vi "globalArrows.vi"() -> ()   [LabVIEW 2020]
panel:
  out "empty":u32[][](array[colorbox])=[[0, 0, 0, 0, 0, 0, 0, 0], [0, 0, 0, 0, 0, 0, 0, 0], [0, 0, 0, 0, 0, 0, 0, 0], [0, 0, 0, 0, 0, 0, 0, 0], [0, 0, 0, 0, 0, 0, 0, 0], [0, 0, 0, 0, 0, 0, 0, 0], [0, 0, 0, 0, 0, 0, 0, 0], [0, 0, 0, 0, 0, 0, 0, 16777222]]
  out "left":u32[][](array[colorbox])=[[0, 0, 0, 0, 0, 0, 0, 0], [0, 0, 6618880, 0, 0, 0, 0, 0], [0, 6618880, 0, 0, 0, 0, 0, 0], [6618880, 6618880, 6618880, 6618880, 6618880, 6618880, 0, 0], [0, 6618880, 0, 0, 0, 0, 0, 0], [0, 0, 6618880, 0, 0, 0, 0, 0], [0, 0, 0, 0, 0, 0, 0, 0], [16777222, 0, 0, 0, 0, 0, 0, 0]]
  out "up":u32[][](array[colorbox])=[[0, 0, 0, 6618880, 0, 0, 0, 16777222], [0, 0, 6618880, 6618880, 6618880, 0, 0, 0], [0, 6618880, 0, 6618880, 0, 6618880, 0, 0], [0, 0, 0, 6618880, 0, 0, 0, 0], [0, 0, 0, 6618880, 0, 0, 0, 0], [0, 0, 0, 6618880, 0, 0, 0, 0], [0, 0, 0, 0, 0, 0, 0, 0], [0, 0, 0, 0, 0, 0, 0, 0]]
  out "down":u32[][](array[colorbox])=[[0, 0, 0, 0, 0, 0, 0, 0], [0, 0, 0, 0, 0, 0, 0, 0], [0, 0, 0, 6618880, 0, 0, 0, 0], [0, 0, 0, 6618880, 0, 0, 0, 0], [0, 0, 0, 6618880, 0, 0, 0, 0], [0, 6618880, 0, 6618880, 0, 6618880, 0, 0], [0, 0, 6618880, 6618880, 6618880, 0, 0, 0], [0, 0, 0, 6618880, 0, 0, 0, 16777222]]
  out "enter":u32[][](array[colorbox])=[[0, 0, 0, 0, 0, 0, 6618880, 0], [0, 0, 6618880, 0, 0, 0, 6618880, 0], [0, 6618880, 0, 0, 0, 0, 6618880, 0], [6618880, 6618880, 6618880, 6618880, 6618880, 6618880, 6618880, 0], [0, 6618880, 0, 0, 0, 0, 0, 0], [0, 16777222, 6618880, 0, 0, 0, 0, 0], [0, 0, 16777222, 0, 0, 0, 0, 0], [0, 0, 0, 0, 0, 0, 0, 16777222]]
  out "right":u32[][](array[colorbox])=[[0, 0, 0, 0, 0, 0, 0, 0], [0, 0, 0, 0, 0, 6618880, 0, 0], [0, 0, 0, 0, 0, 0, 6618880, 0], [0, 0, 6618880, 6618880, 6618880, 6618880, 6618880, 6618880], [0, 0, 0, 0, 0, 0, 6618880, 0], [0, 0, 0, 0, 0, 6618880, 0, 0], [0, 0, 0, 0, 0, 0, 0, 0], [0, 0, 0, 0, 0, 0, 0, 16777222]]
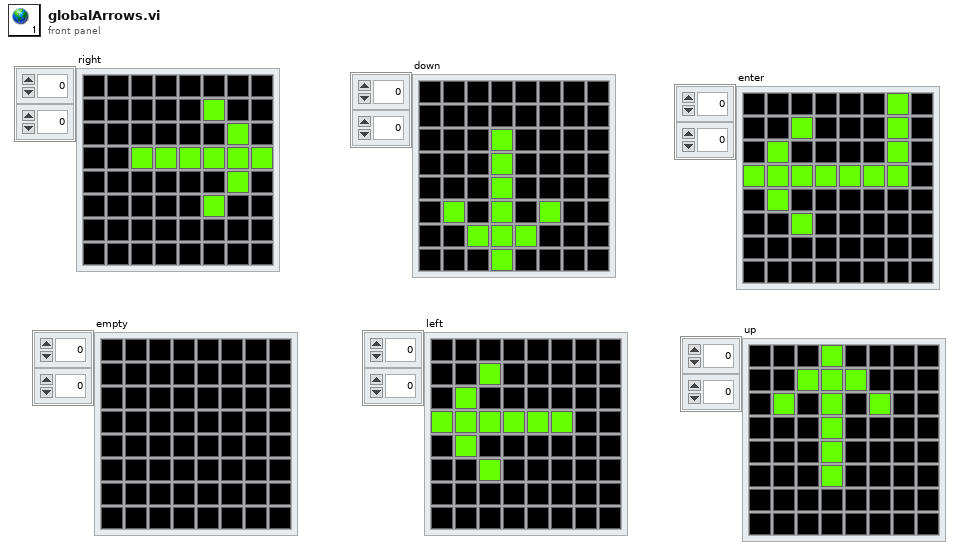
[diagram p1: front panel]
diagram:
